vi "Initialize Configuration Channels.vi"(8 "error in (no error)":errorcluster, 10 "Configuration Channels":string[](array[string]), 11 "Session In":T1) -> (0 "error out":errorcluster, 3 "Session out":T1)   [LabVIEW 2020, in "%DEVICE% Messaging.lvlib" / "Consumer.lvclass"]
uses:
  Consumer.lvclass
  Session Type.ctl
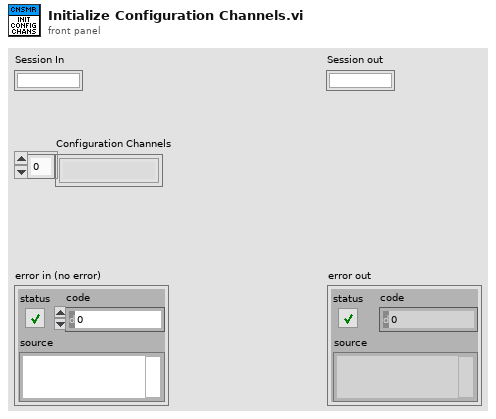
[diagram p1: front panel]
types:
  T1 = typedef "%DEVICE% Messaging.lvlib/Consumer.lvclass/Session Type.ctl" = picture
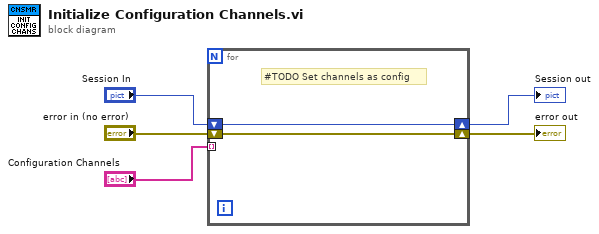
[diagram p0: block diagram]
diagram:
  n1 = for {
    shift-right: [w6] -> w5
    shift-left: "error in (no error)" -> [w6]
    shift-right: [w7] -> w1
    shift-left: "Session In" -> [w7]
    tunnel: "Configuration Channels" -> [_] mode=indexing
    # "#TODO Set channels as config"
  }
  "error out" <- w5
  "Session out" <- w1
